vi "niFpgaBFGroupRegular.vi"(1 "mult output type":fxp<+/-,18,2> format="%.17g", 2 "bf bullet type":fxp<+/-,16,1> format="%.16g", 5 "bf data in":T1 {"x_r" format="%.16g"; "x_i" format="%.16g"; "y_r" format="%.16g"; "y_i" format="%.16g"}, 7 "stage switch in":bool, 9 "tf index in":fxp<+,7,7>) -> (6 "bf data out":T1 {"x_r" format="%.16g"; "x_i" format="%.16g"; "y_r" format="%.16g"; "y_i" format="%.16g"}, 8 "stage switch out":bool, 10 "tf index out":fxp<+,7,7>)   [LabVIEW 2017]
uses:
  <vilib>/rvi/Analysis/measure/FFT/supportingXNodes/permutation/XNode/niFpgaFFTPermutation.xnode
  <vilib>/rvi/FXPMathLib/basic elements/FxpDiscreteDelay/XNode/nifxpmath_DiscreteDelay.xnode
  <vilib>/rvi/Analysis/measure/FFT/supportingXNodes/butterfly/XNode/niFpgaFFTDIFButterfly.xnode
  <vilib>/rvi/FXPMathLib/FxpMul/XNode/nifxpmath_Multiplier.xnode
  <vilib>/rvi/FXPMathLib/sim/FxpSim.dll
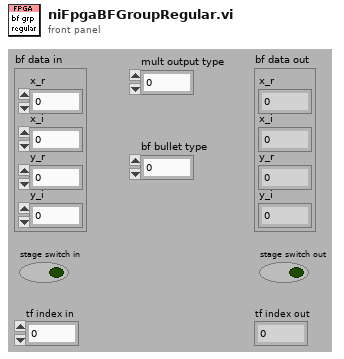
[diagram p1: front panel]
types:
  T1 = cluster{"x_r":fxp<+/-,16,1>, "x_i ":fxp<+/-,16,1>, "y_r ":fxp<+/-,16,1>, "y_i ":fxp<+/-,16,1>}
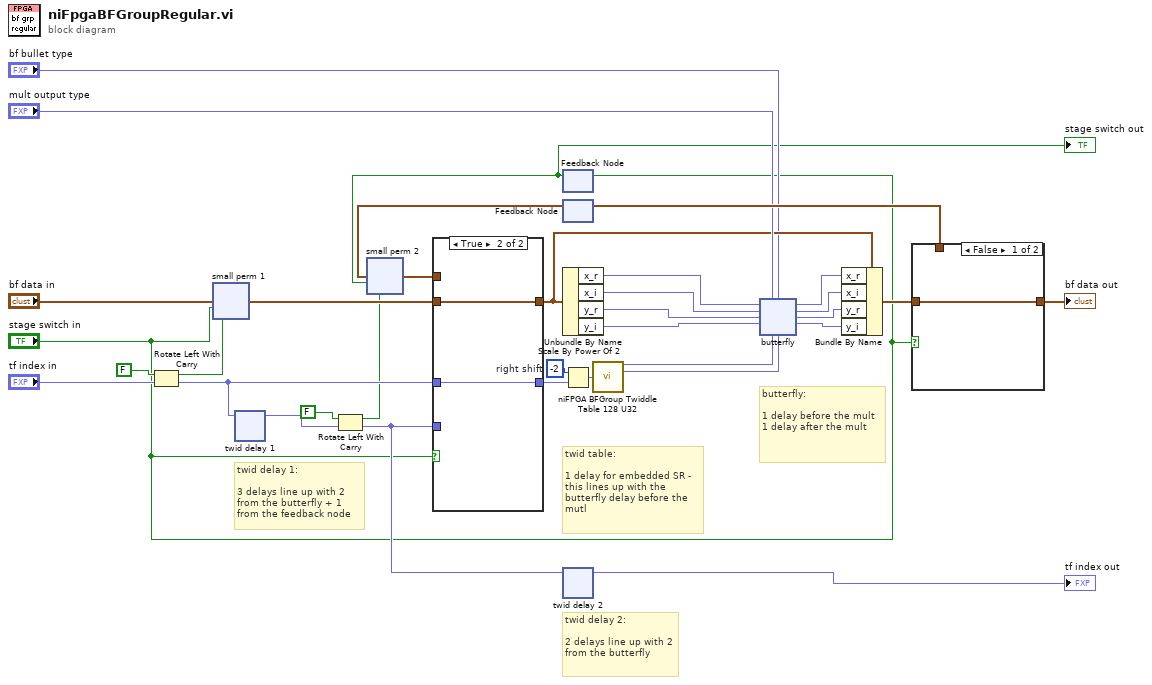
[diagram p0: block diagram]
diagram:
  w2 = -2  # right shift
  # "twid delay 2:\n\n2 delays line up with 2 from the butterfly"
  # "twid delay 1:\n\n3 delays line up with 2 from the butterfly + 1 from the feedback node"
  # "twid table:\n\n1 delay for embedded SR - this lines up with the butterfly delay before the mutl"
  # "butterfly: \n\n1 delay before the mult\n1 delay after the mult"
  n1 = Rotate Left With Carry(2:"tf index in", 3:FALSE ("carry")) -> (0:w17:fxp<+,7,7>, 1:w11:bool)
  n2 = xnode "small perm 1"("bf data in"="bf data in", "stage switch"="stage switch in", "perm switch"=w11) -> ("bf data out"=w9:T1)
  n3 = xnode "twid delay 1"("D"=w17) -> ("Q"=w15:fxp<+,7,7>)
  n4 = Rotate Left With Carry(2:w15, 3:FALSE ("carry")) -> (0:w14:fxp<+,7,7>, 1:w5:bool)
  n5 = feedback-in #1("stage switch in") -> ()
  n6 = feedback #1() -> (w6:bool)  [unwired: 1 out]
  "stage switch out" <- w6
  n7 = feedback #2() -> (w7:T1)  [unwired: 1 out]
  n8 = xnode "small perm 2"("bf data in"=w7, "stage switch"=w6, "perm switch"=w5) -> ("bf data out"=w8:T1)
  n9 = case shown="True" "stage switch in" {
    tunnel: [w36 w38] -> w21
    tunnel: w9 -> [_ w38]
    tunnel: w8 -> [w36 _]
    tunnel: w14 -> [w35 _]
    tunnel: [w35 w37] -> w4
    tunnel: w17 -> [_ w37]
    frame False {
    }
    frame True {
    }
  }
  n10 = Unbundle By Name(w21) -> ("x_r"=w31:fxp<+/-,16,1>, "x_i"=w30:fxp<+/-,16,1>, "y_r"=w29:fxp<+/-,16,1>, "y_i"=w28:fxp<+/-,16,1>)
  n11 = Scale By Power Of 2(n=w2, x=w4) -> (x*2^n=w3:fxp<+,7,7>)
  n12 = xnode "twid delay 2"("D"=w14) -> ("Q"=→"tf index out":fxp<+,7,7>)
  n13 = call <vilib>:"niFPGA BFGroup Twiddle Table 128 U32.vi"("address"=w3) -> ("twid real"=w20:fxp<+/-,17,2>, "twid imag"=w1:fxp<+/-,17,2>)  [unwired: 13 out]
  n14 = xnode "butterfly"("x_r"=w31, "x_i"=w30, "y_r"=w29, "y_i"=w28, "tf_r"=w20, "tf_i"=w1, "mult output type"="mult output type", "bf bullet type"="bf bullet type") -> ("x_out_r"=w27:fxp<+/-,16,1>, "x_out_i"=w26:fxp<+/-,16,1>, "y_out_r"=w25:fxp<+/-,16,1>, "y_out_i"=w24:fxp<+/-,16,1>)  [unwired: 1 in]
  n15 = Bundle By Name(cluster=w21, "x_r"=w27, "x_i"=w26, "y_r"=w25, "y_i"=w24) -> (w23:T1)
  n16 = case shown="False" "stage switch in" {
    tunnel: [_ w40] -> w34
    tunnel: w23 -> [w39 w40]
    tunnel: [w39 _] -> w33
    frame False {
    }
    frame True {
    }
  }
  "bf data out" <- w33
  n17 = feedback-in #2(w34) -> ()
